vi "M26C_SR830.vi"() -> ()   [LabVIEW 2024]
uses:
  <instrlib>/Stanford Research 830/Stanford Research 830.lvlib
  <instrlib>/Stanford Research 830/Public/Data/Read (All Parameters).vi
panel:
  in  "Setpoint":dbl=300.0
  in  "Stop Program Loop":bool
  out "File I/O Error Out":errorcluster
  out "Dup path":path
  in  "<File Name>.txt (Don't add extension)":string
  in  "Data Save Path:":path=path "C:/Users"
  out "Temp & Time":cluster{"Y":dbl[], "Y":dbl[]}[](graph)
  out "R & Time":cluster{"Y":dbl[], "Y":dbl[]}[](graph)
  out "Theta & Time":cluster{"Y":dbl[], "Y":dbl[]}[](graph)
  in  "Minimum Loop \nTime (milliseconds)":u32=100
  in  "Temp Input Channel":u8(ring) items=["ChA", "ChB"]
  out "Temperature":dbl format="%.2f"
  in  "I":sgl=60.0 min=0 step=1 format="%.2f"
  in  "D":sgl format="%.2f"
  in  "P":sgl=2.0 format="%.2f"
  in  "Output":u8(ring) items=["Loop 1", "Loop 2", "Loop 3", "Loop 4"]
  in  "Serial Configuration":cluster{"Baud Rate":u32}={"Baud Rate"=9600} {"Baud Rate" items=["300"=300, "600"=600, "1200"=1200, "2400"=2400, "4800"=4800, "9600"=9600, "19200"=19200]}
  in  "Reset":bool=TRUE
  in  "M26C Temperature Controller\n resource name":refnum<visa-resource-name>="tcpip0::192.168.1.5::5000::SOCKET"
  in  "SR830 Lock-in Amplifier\nresource name":refnum<visa-resource-name>
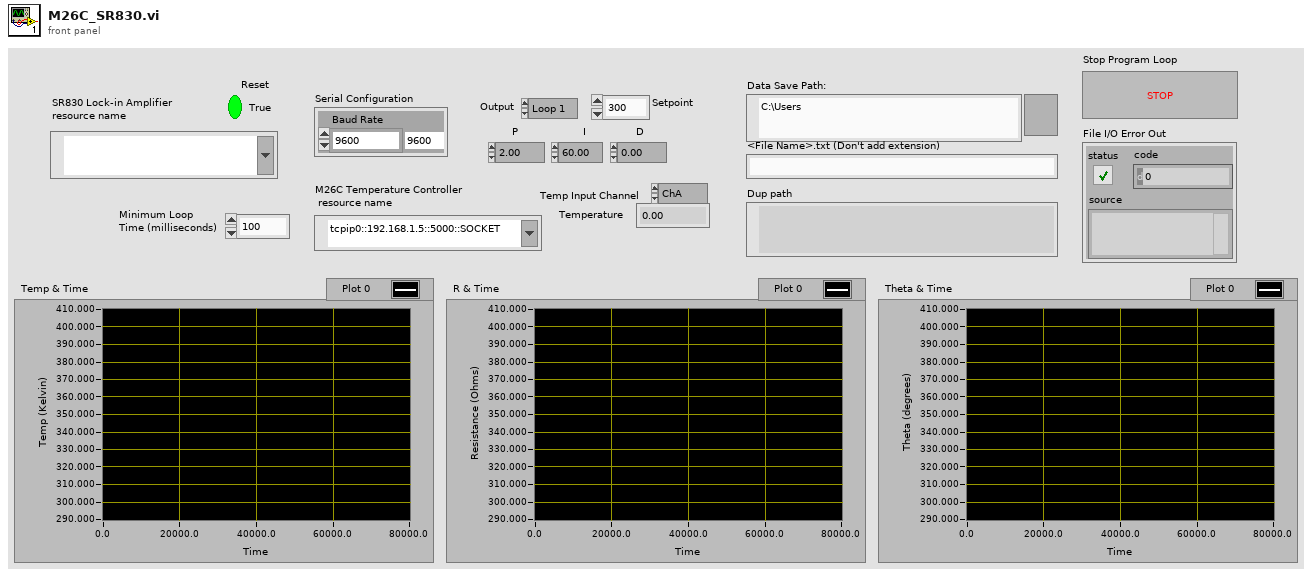
[diagram p1: front panel]
types:
  T1 = enum16{"open", "replace", "create", "open or create", "replace or create", "replace or create with confirmation"}
  T2 = cluster{"X-Value":dbl, "Y-Value":dbl, "R-Value":dbl, "Theta-Value":dbl, "Aux In 1 Value":dbl, "Aux In 2 Value":dbl, "Aux In 3 Value":dbl, "Aux In 4 Value":dbl, "Reference Frequency":dbl, "Channel 1 Display":dbl, "Channel 2 Display":dbl}
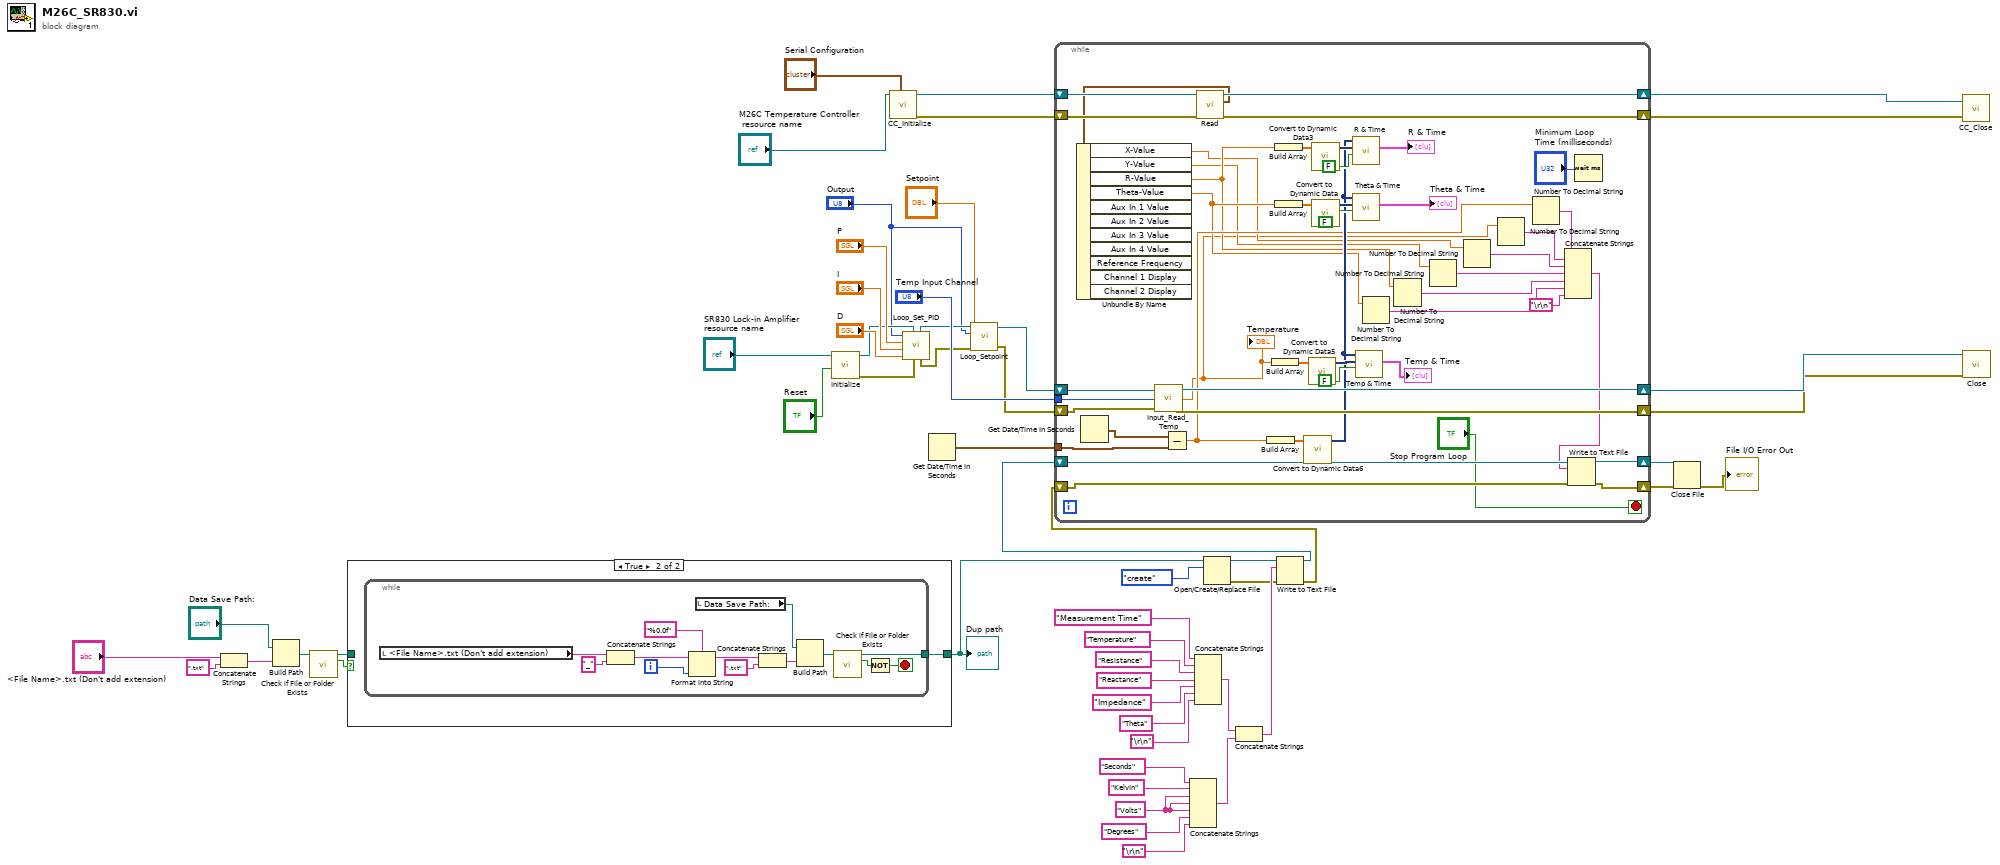
[diagram p0: block diagram]
diagram:
  w19 = "Volts" ("string")
  n1 = Concatenate Strings("<File Name>.txt (Don't add extension)", ".txt") -> (w35:string)
  n2 = Build Path(base path="Data Save Path:", name or relative path=w35) -> (appended path=w34:path)
  n3 = call <vilib>:"Check if File or Folder Exists.vi"("path"=w34) -> ("file or folder exists?"=w33:bool, "dup path"=w32:path)  [unwired: 8 in, 1 out]
  n4 = case shown="True" w33 {
    tunnel: [w55 w56] -> w16
    tunnel: w32 -> [w55 _]
    frame False {
    }
    frame True {
      n5 = while {
        tunnel: [w62] -> w56
        i -> [w66]
        stop <- w68 stop-if-true
        n6 = local read "<File Name>.txt (Don't add extension)"() -> (w58:string)
        n7 = Concatenate Strings(w58, "_" ("string")) -> (w61:string)
        n8 = Format Into String(format string="%0.0f", initial string=w61, w66) -> (resulting string=w65:string)  [unwired: 1 in, 1 out]
        n9 = local read "Data Save Path:"() -> (w57:path)
        n10 = Concatenate Strings(w65, ".txt") -> (w64:string)
        n11 = Build Path(base path=w57, name or relative path=w64) -> (appended path=w63:path)
        n12 = call <vilib>:"Check if File or Folder Exists.vi"("path"=w63) -> ("file or folder exists?"=w69:bool, "dup path"=w62:path)  [unwired: 8 in, 1 out]
        n13 = Not(x=w69) -> (.not. x?=w68:bool)
      }
    }
  }
  "Dup path" <- w16
  n14 = call <instrlib>:"Initialize.vi"("Reset (True)"="Reset", "VISA resource name"="SR830 Lock-in Amplifier\nresource name") -> ("error out"=w46:errorcluster, "VISA resource name out"=w47:refnum<visa-resource-name>)  [unwired: 8 in]
  n15 = call <instrlib>:"CC_Initialize.vi"("Serial Configuration"="Serial Configuration", "VISA resource name"="M26C Temperature Controller\n resource name") -> ("error out"=w40:errorcluster, "VISA resource name out"=w42:refnum<visa-resource-name>)  [unwired: 8 in]
  n16 = call <instrlib>:"Loop_Set_PID.vi"("error in (no error)"=w46, "VISA In"=w47, "D"="D", "I"="I", "P"="P", "Loop"="Output") -> ("error out"=w4:errorcluster, "VISA Out"=w6:refnum<visa-resource-name>)  [unwired: 4 in]
  n17 = Get Date/Time In Seconds() -> (seconds since 1Jan1904=w38:timestamp)
  n18 = call <instrlib>:"Loop_Setpoint.vi"("VISA in"=w6, "Loop"="Output", "Setpoint"="Setpoint", "error in"=w4) -> ("VISA out"=w5:refnum<visa-resource-name>, "ErrorOut"=w3:errorcluster)  [unwired: 1 in, 1 out]
  n19 = Concatenate Strings("Seconds" ("string"), "Kelvin" ("string"), w19, w19, w19, "Degrees" ("string"), "\r\n") -> (w17:string)
  n20 = Concatenate Strings("Measurement Time" ("string"), "Temperature" ("string"), "Resistance" ("string"), "Reactance" ("string"), "Impedance" ("string"), "Theta" ("string"), "\r\n") -> (w30:string)
  n21 = Open/Create/Replace File(file path (use dialog)=w16, operation (0:open)=T1."create") -> (refnum out=w15:refnum<file>, error out=w13:errorcluster)  [unwired: 4 in, 1 out]
  n22 = Concatenate Strings(w30, w17) -> (w14:string)
  n23 = Write to Text File(file (use dialog)=w15, text=w14, error in=w13) -> (refnum out=w12:refnum<file>, error out=w11:errorcluster)  [unwired: 1 in, 1 out]
  n24 = while {
    tunnel: "Temp Input Channel" -> [w115]
    shift-right: [w113] -> w44
    shift-left: w5 -> [w114]
    shift-right: [w111] -> w43
    shift-left: w3 -> [w112]
    shift-right: [w108] -> w41
    shift-left: w42 -> [w109]
    shift-right: [w106] -> w39
    shift-left: w40 -> [w107]
    tunnel: w38 -> [w100]
    shift-right: [w85] -> w10
    shift-left: w12 -> [w88]
    shift-right: [w86] -> w9
    shift-left: w11 -> [w87]
    stop <- "Stop Program Loop" stop-if-true
    n25 = Get Date/Time In Seconds() -> (seconds since 1Jan1904=w101:timestamp)
    n26 = call <instrlib>:"Input_Read_Temp.vi"("error in (no error)"=w112, "Input"=w115, "VISA In"=w114) -> ("error out"=w111:errorcluster, "Temperature"=w71:dbl, "VISA Out"=w113:refnum<visa-resource-name>)
    "Temperature" <- w71
    n27 = Subtract(x=w101, y=w100) -> (x-y=w76:dbl)
    n28 = call-poly <instrlib>:"Read.vi"("error in (no error)"=w107, "VISA resource name"=w109) -> ("error out"=w106:errorcluster, "Parameter Values"=w83:T2, "VISA resource name out"=w108:refnum<visa-resource-name>)  [unwired: 7 in]
    n29 = Unbundle By Name(w83) -> ("X-Value"=w72:dbl, "Y-Value"=w73:dbl, "R-Value"=w74:dbl, "Theta-Value"=w75:dbl)  [unwired: 7 out]
    n30 = Build Array(w76) -> (w95:dbl[])
    n31 = Build Array(w71) -> (w92:dbl[])
    n32 = Build Array(w74) -> (w97:dbl[])
    n33 = Build Array(w75) -> (w103:dbl[])
    n34 = call "Convert to Dynamic Data6"("Array"=w95) -> ("Dynamic Data Type"=w90:dynamicdata)  [unwired: 3 in]
    n35 = call "Convert to Dynamic Data5"("Array"=w92) -> ("Dynamic Data Type"=w93:dynamicdata)  [unwired: 3 in]
    n36 = call "Convert to Dynamic Data3"("Array"=w97) -> ("Dynamic Data Type"=w98:dynamicdata)  [unwired: 3 in]
    n37 = call "Convert to Dynamic Data"("Array"=w103) -> ("Dynamic Data Type"=w104:dynamicdata)  [unwired: 3 in]
    n38 = call "R & Time"("Reset"=FALSE, "Y Input"=w98, "X Input"=w90) -> ("XY Graph"=→"R & Time":cluster{"X":dbl[], "Y":dbl[]}[])  [unwired: 7 in, 1 out]
    n39 = call "Theta & Time"("Reset"=FALSE, "Y Input"=w104, "X Input"=w90) -> ("XY Graph"=→"Theta & Time":cluster{"X":dbl[], "Y":dbl[]}[])  [unwired: 7 in, 1 out]
    n40 = call "Temp & Time"("Reset"=FALSE, "Y Input"=w93, "X Input"=w90) -> ("XY Graph"=→"Temp & Time":cluster{"X":dbl[], "Y":dbl[]}[])  [unwired: 7 in, 1 out]
    n41 = Number To Decimal String(number=w75) -> (decimal integer string=w82:string)  [unwired: 1 in]
    n42 = Number To Decimal String(number=w74) -> (decimal integer string=w81:string)  [unwired: 1 in]
    n43 = Number To Decimal String(number=w73) -> (decimal integer string=w80:string)  [unwired: 1 in]
    n44 = Number To Decimal String(number=w72) -> (decimal integer string=w79:string)  [unwired: 1 in]
    n45 = Number To Decimal String(number=w71) -> (decimal integer string=w78:string)  [unwired: 1 in]
    n46 = Number To Decimal String(number=w76) -> (decimal integer string=w77:string)  [unwired: 1 in]
    n47 = Concatenate Strings(w77, w78, w79, w80, w81, w82, "\r\n") -> (w84:string)
    n48 = Write to Text File(file (use dialog)=w88, text=w84, error in=w87) -> (refnum out=w85:refnum<file>, error out=w86:errorcluster)  [unwired: 1 in, 1 out]
    n49 = Wait (ms)(milliseconds to wait="Minimum Loop \nTime (milliseconds)") -> ()  [unwired: 1 out]
  }
  n50 = Close File(refnum=w10, error in=w9) -> (error out=→"File I/O Error Out":errorcluster)  [unwired: 1 out]
  n51 = call <instrlib>:"CC_Close.vi"("error in (no error)"=w39, "VISA In"=w41) -> ()  [unwired: 1 in, 1 out]
  n52 = call <instrlib>:"Close.vi"("error in (no error)"=w43, "VISA resource name"=w44) -> ()  [unwired: 9 in, 1 out]
